vi "Convert Old CAN Log to XNET.vi"() -> ()   [LabVIEW 2014]
uses:
  <vilib>/RioEmbeddedCAN/RioEmbeddedCAN.llb/CANFrameControl.ctl
panel:
  in  "New File path":path
  in  "Source":path=path "C:/Data for Processing/150215 132046.tdms"
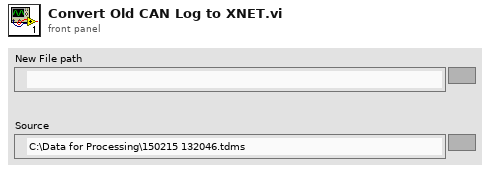
[diagram p1: front panel]
types:
  T1 = enum16{"big-endian, network order", "native, host order", "little-endian"}
  T2 = enum16{"open", "open or create", "create or replace", "create", "open (read-only)"}
  T3 = typedef "CANFrameControl.ctl" = cluster{"identifier":u32, "extended?":bool, "type":u8, "payload":u8[]}
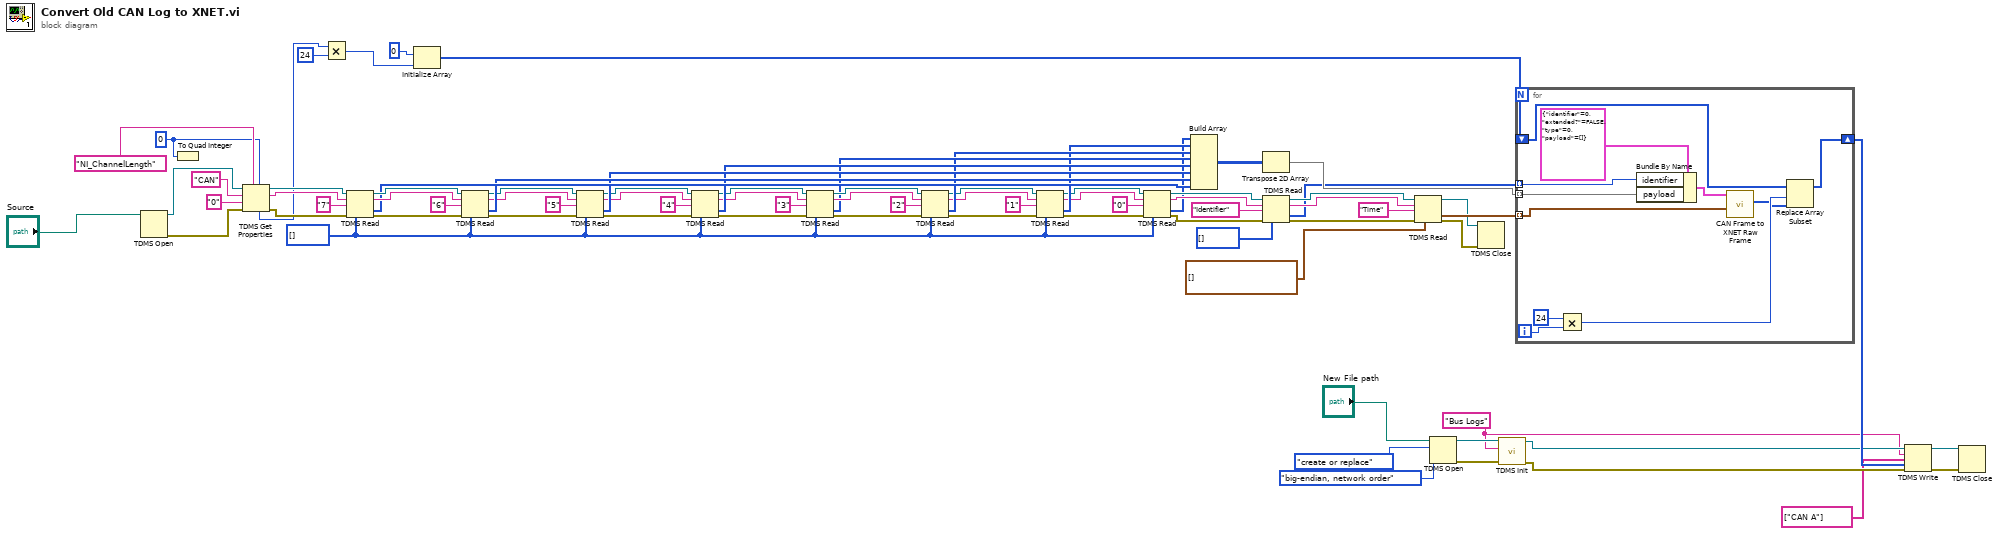
[diagram p0: block diagram]
diagram:
  w6 = "Bus Logs" ("group name")
  w25 = u8[] []
  w75 = u64 0 ("data type")
  n1 = TDMS Open(11:"Source") -> (0:w80:errorcluster, 3:w81:refnum<k34>)  [unwired: 6 in]
  n2 = To Quad Integer(1:w75) -> ()  [unwired: 1 out]
  n3 = TDMS Get Properties(5:w75, 7:"NI_ChannelLength" ("property name"), 8:w80, 9:"0" ("channel name"), 10:"CAN" ("group name"), 11:w81) -> (0:w73:errorcluster, 2:w72:string, 3:w74:refnum<k34>, 4:w17:u64)  [unwired: 2 out]
  n4 = Multiply(x=w17, y=u64 24) -> (x*y=w15:u64)
  n5 = TDMS Read(0:w74, 5:w72, 7:"7" ("channel name(s) in"), 11:w73, 12:w25) -> (4:w70:refnum<k34>, 6:w68:string, 10:w66:u8[], 15:w69:errorcluster)  [unwired: 3 in, 2 out]
  n6 = Initialize Array(u8 0, w15) -> (w13:u8[])
  n7 = TDMS Read(0:w70, 5:w68, 7:"6" ("channel name(s) in"), 11:w69, 12:w25) -> (4:w64:refnum<k34>, 6:w62:string, 10:w65:u8[], 15:w63:errorcluster)  [unwired: 3 in, 2 out]
  n8 = TDMS Read(0:w64, 5:w62, 7:"5" ("channel name(s) in"), 11:w63, 12:w25) -> (4:w59:refnum<k34>, 6:w58:string, 10:w60:u8[], 15:w56:errorcluster)  [unwired: 3 in, 2 out]
  n9 = TDMS Read(0:w59, 5:w58, 7:"4" ("channel name(s) in"), 11:w56, 12:w25) -> (4:w54:refnum<k34>, 6:w52:string, 10:w55:u8[], 15:w53:errorcluster)  [unwired: 3 in, 2 out]
  n10 = TDMS Read(0:w54, 5:w52, 7:"3" ("channel name(s) in"), 11:w53, 12:w25) -> (4:w50:refnum<k34>, 6:w48:string, 10:w45:u8[], 15:w49:errorcluster)  [unwired: 3 in, 2 out]
  n11 = TDMS Read(0:w50, 5:w48, 7:"2" ("channel name(s) in"), 11:w49, 12:w25) -> (4:w27:refnum<k34>, 6:w21:string, 10:w44:u8[], 15:w26:errorcluster)  [unwired: 3 in, 2 out]
  n12 = TDMS Read(0:w27, 5:w21, 7:"1" ("channel name(s) in"), 11:w26, 12:w25) -> (4:w20:refnum<k34>, 6:w18:string, 10:w24:u8[], 15:w19:errorcluster)  [unwired: 3 in, 2 out]
  n13 = TDMS Read(0:w20, 5:w18, 7:"0" ("channel name(s) in"), 11:w19, 12:w25) -> (4:w43:refnum<k34>, 6:w41:string, 10:w23:u8[], 15:w42:errorcluster)  [unwired: 3 in, 2 out]
  n14 = Build Array(w23, w24, w44, w45, w55, w60, w65, w66) -> (w33:u8[][])
  n15 = Transpose 2D Array(2D array=w33) -> (transposed array=w32:u8[][])
  n16 = TDMS Read(0:w43, 5:w41, 7:"Identifier" ("channel name(s) in"), 11:w42, 12:u32[] []) -> (4:w38:refnum<k34>, 6:w36:string, 10:w30:u32[], 15:w37:errorcluster)  [unwired: 3 in, 2 out]
  n17 = TDMS Read(0:w38, 5:w36, 7:"Time" ("channel name(s) in"), 11:w37, 12:timestamp[] []) -> (4:w29:refnum<k34>, 10:w31:timestamp[], 15:w28:errorcluster)  [unwired: 3 in, 3 out]
  n18 = TDMS Open(9:T1."big-endian, network order" ("byte order (2:little-endian)"), 10:T2."create or replace" ("operation (0:open)"), 11:"New File path") -> (0:w10:errorcluster, 3:w11:refnum<k34>)  [unwired: 4 in]
  n19 = TDMS Close(8:w28, 11:w29) -> ()  [unwired: 2 out]
  n20 = call "TDMS Init.vi"("error in (no error)"=w10, "group name"=w6, "tdms file"=w11) -> ("error out"=w7:errorcluster, "tdms file out"=w8:refnum<k34>)  [unwired: 7 in]
  n21 = for {
    tunnel: w32 -> [w91] mode=indexing
    tunnel: w31 -> [w88] mode=indexing
    tunnel: w30 -> [w90] mode=indexing
    shift-right: [w86] -> w9
    shift-left: w13 -> [w87]
    i -> [w85]
    n22 = Multiply(x=24, y=w85) -> (x*y=w83:i32)
    n23 = Bundle By Name(cluster=T3 {"identifier"=0, "extended?"=FALSE, "type"=0, "payload"=[]} ("CAN frame"), "identifier"=w90, "payload"=w91) -> (w89:T3)
    n24 = call "CAN Frame to XNET Raw Frame.vi"("timestamp"=w88, "CAN frame"=w89) -> ("Raw Frame"=w82:u8[])  [unwired: 9 in]
    n25 = Replace Array Subset(array=w87, new element=w82, index=w83) -> (w86:u8[])
  }
  n26 = TDMS Write(0:w8, 5:w6, 7:string[] ["CAN A"] ("channel name(s) in (Untitled)"), 9:w9, 11:w7) -> (4:w4:refnum<k34>, 15:w3:errorcluster)  [unwired: 1 in, 2 out]
  n27 = TDMS Close(8:w3, 11:w4) -> ()  [unwired: 2 out]
